vi "Setup.vi"(11 "Hello World Event in":refnum<class "Hello World Event.lvclass">) -> (3 "Hello World Event out":refnum<class "Hello World Event.lvclass">)   [LabVIEW 2021, in "Hello World Event.lvlib" / "Hello World Event.lvclass"]
uses:
  Hello World Event.lvclass
  Hello World Event.lvclass/Hello World Event.ctl
  Actor/Event Actor/Event Actor.lvclass
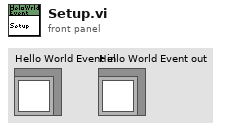
[diagram p1: front panel]
types:
  T1 = enum32{"Invalid", "Standard", "Closed", "Hidden", "Minimized", "Maximized"}
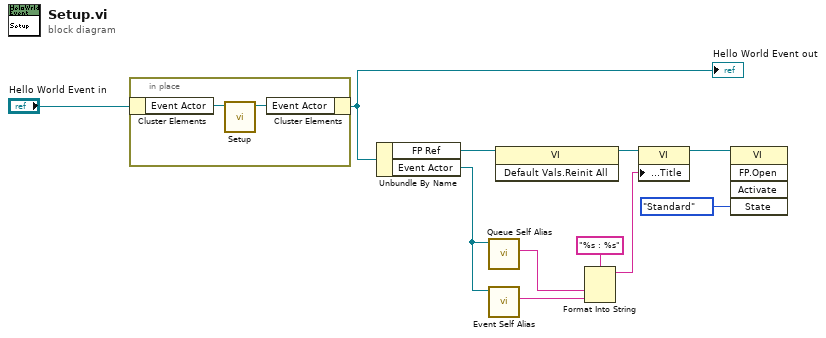
[diagram p0: block diagram]
diagram:
  n1 = in-place {
    n2 = in-place-cluster #1("Hello World Event in") -> ("Event Actor"=w13:refnum<class "Event Actor.lvclass">)
    n3 = call-dynamic "Setup.vi"("Setup in"=w13) -> ("Setup out"=w12:refnum<class "Event Actor.lvclass">)  [unwired: 10 in]
    n4 = in-place-cluster #1("Event Actor"=w12) -> (w6:refnum<class "Hello World Event.lvclass">)
  }
  "Hello World Event out" <- w6
  n5 = Unbundle By Name(w6) -> ("FP Ref"=w9:refnum<vi>, "Event Actor"=w5:refnum<class "Event Actor.lvclass">)
  n6 = call-dynamic "Queue Self Alias.vi"("Actor in"=w5) -> ("Queue Self Alias"=w4:string)  [unwired: 10 in]
  n7 = call-dynamic "Event Self Alias.vi"("Actor in"=w5) -> ("Event Self Alias"=w2:string)  [unwired: 10 in]
  n8 = invoke class="VI" method="Default Vals.Reinit All"(reference=w9) -> (reference out=w8:refnum<vi>)  [unwired: 2 in, 2 out]
  n9 = Format Into String(format string="%s : %s", w4, w2) -> (resulting string=w3:string)  [unwired: 2 in, 1 out]
  n10 = property class="VI"(reference=w8, "Front Panel.Title"=w3) -> (reference out=w7:refnum<vi>)  [unwired: 1 in, 1 out]
  n11 = invoke class="VI" method="FP.Open"(reference=w7, "State"=T1."Standard") -> ()  [unwired: 3 in, 5 out]
